vi "Source_Live_Control_Manual.vi"() -> ()   [LabVIEW 2022 SP3]
panel:
  in  "Source Live":bool
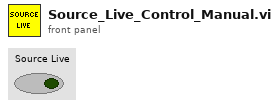
[diagram p1: front panel]
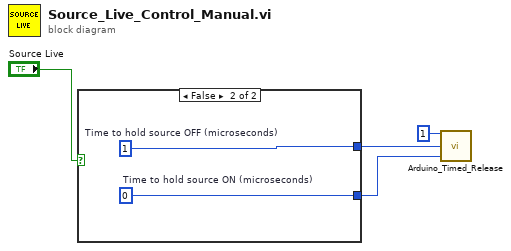
[diagram p0: block diagram]
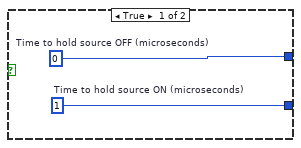
[diagram p2: hidden frame]
diagram:
  n1 = case shown="False" "Source Live" {
    tunnel: [w6 w8] -> w3
    tunnel: [w5 w7] -> w2
    frame True {
      w5 = u32 0  # Time to hold source OFF (microseconds)
      w6 = u32 1  # Time to hold source ON (microseconds)
    }
    frame False {
      w7 = u32 1  # Time to hold source OFF (microseconds)
      w8 = u32 0  # Time to hold source ON (microseconds)
    }
  }
  n2 = call "Arduino_Timed_Release.vi"("Time to hold source ON (microseconds)"=w3, "Time to hold source OFF (microseconds)"=w2, "Number of cycles"=u16 1) -> ()  [unwired: 2 out]
